vi "Open Swerve Drive.vi"   [LabVIEW 2014]
doc: "Opens references and stores refnums for all swerve drive motors, steering encoders, and gyro(s). The gyros are opened using the Apple Pi gyro library. If you wish to use the normal (WPILib) gyro code, then remove the open blocks from inside this VI."
uses:
  <vilib>/Rock Robotics/SystemInterfaces/DIO/FPGA_DIOPWMChannel.ctl
  <vilib>/Rock Robotics/SystemInterfaces/AI/FPGA_AIChannel.ctl
  <vilib>/Rock Robotics/WPI/MotorControl/WPI_MotorControlOpen Talon.vi
  Global Variables/Refnum Names.vi
types:
  T1 = typedef "FPGA_AIChannel.ctl" = enum8{"AI 0", "AI 1", "AI 2", "AI 3", "AI MXP 0", "AI MXP 1", "AI MXP 2", "AI MXP 3", "Invalid"}
  T2 = typedef "FPGA_DIOPWMChannel.ctl" = enum8{"PWM 0", "PWM 1", "PWM 2", "PWM 3", "PWM 4", "PWM 5", "PWM 6", "PWM 7", "PWM 8", "PWM 9", "PWM MXP 0", "PWM MXP 1", "PWM MXP 2", "PWM MXP 3", "PWM MXP 4", "PWM MXP 5", "PWM MXP 6", "PWM MXP 7", "PWM MXP 8", "PWM MXP 9", "Invalid"}
  T3 = typedef "WPI_MotorControlDeviceRef.ctl" = cluster{"DeviceStatus":errorcluster, "Type":T4, "PWM":cluster{"Controller":T5, "PWM Channel":T2, "DeadBand":T6}, "CAN":cluster{"Device Number":u8, "Control Mode":T7, "Semaphore":T8, "Max Vout":dbl, "TalonSRX Control Mode":T9}, "Invert":bool, "TransformRef":T10, "InvTransformRef":T10}
  T4 = typedef "WPI_MotorControlType.ctl" = enum16{"PWM", "CAN", "CANTalonSRX"}
  T5 = typedef "FPGA_TypedefDigitalModule.ctl" = enum16{"Controller 1"}
  T6 = typedef "WPI_PWMDeadband.ctl" = cluster{"Name":string, "maxPositivePwm":i32, "minPositivePwm":i32, "centerPwm":i32, "maxNegativePwm":i32, "minNegativePwm":i32, "angularRange":u16}
  T7 = typedef "WPI_CANJaguar_ControlMode.ctl" = enum8{"Percent VBus", "Current", "Speed", "Position", "Voltage"}
  T8 = typedef "Semaphore RefNum" = refnum<k1>
  T9 = typedef "WPI_CANTalonSRX_APIControlMode.ctl" = enum8{"Percent VBus", "Speed", "Position", "Slave", "Unchanged / Invalid"}
  T10 = typedef "WPI_PWMTransform_ConPane.ctl" = refnum<vi>
  T11 = typedef "Swerve Sensors DevRef.ctl" = cluster{"Front Right Wheel":T12, "Front Left Wheel":T12, "Rear Right Wheel":T12, "Rear Left Wheel":T12}
  T12 = typedef "WPI_AnalogChannelDevRef.ctl" = cluster{"DevStatus":errorcluster, "Controller":T13, "Analog Channel":T1}
  T13 = typedef "FPGA_TypedefAnalogModule.ctl" = enum16{"Controller 1"}
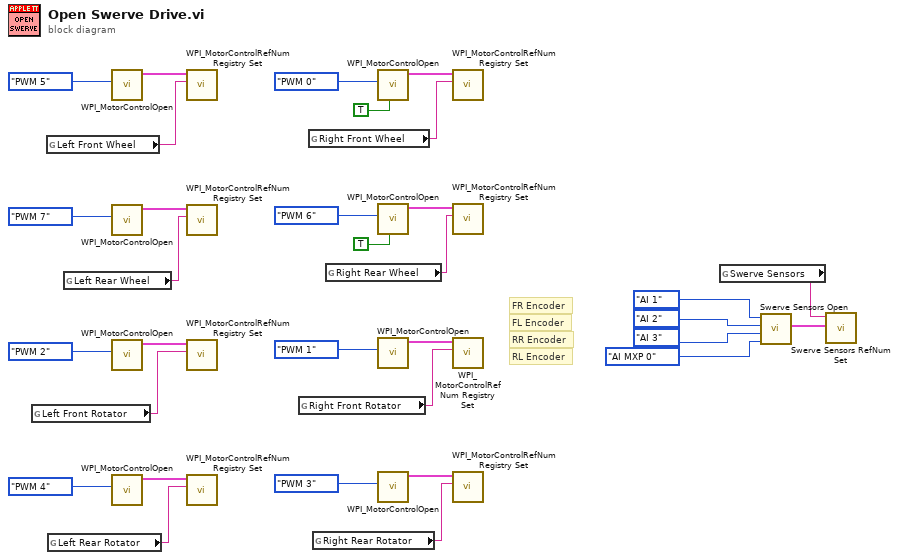
[diagram p0: block diagram]
diagram:
  # "RL Encoder"
  # "RR Encoder"
  # "FL Encoder"
  # "FR Encoder"
  n1 = global read "Refnum Names.vi" "Left Front Rotator"() -> (w7:string)
  n2 = global read "Refnum Names.vi" "Left Front Wheel"() -> (w11:string)
  n3 = global read "Refnum Names.vi" "Left Rear Rotator"() -> (w5:string)
  n4 = global read "Refnum Names.vi" "Left Rear Wheel"() -> (w9:string)
  n5 = call-poly <vilib>:"WPI_MotorControlOpen.vi"("PWM Channel"=FPGA_DIOPWMChannel."PWM 5" ("BL Wheel")) -> ("MotorControlDeviceRef"=w32:T3)  [unwired: 9 in, 1 out]
  n6 = call-poly <vilib>:"WPI_MotorControlOpen.vi"("PWM Channel"=FPGA_DIOPWMChannel."PWM 7" ("BL Spin")) -> ("MotorControlDeviceRef"=w29:T3)  [unwired: 9 in, 1 out]
  n7 = call-poly <vilib>:"WPI_MotorControlOpen.vi"("PWM Channel"=FPGA_DIOPWMChannel."PWM 2" ("BR Wheel")) -> ("MotorControlDeviceRef"=w28:T3)  [unwired: 9 in, 1 out]
  n8 = call-poly <vilib>:"WPI_MotorControlOpen.vi"("PWM Channel"=FPGA_DIOPWMChannel."PWM 4" ("BR Spin")) -> ("MotorControlDeviceRef"=w25:T3)  [unwired: 9 in, 1 out]
  n9 = call <vilib>:"WPI_MotorControlRefNum Registry Set.vi"("refnum name"=w11, "MotorControlDevRef"=w32) -> ()  [unwired: 8 in, 2 out]
  n10 = call <vilib>:"WPI_MotorControlRefNum Registry Set.vi"("refnum name"=w9, "MotorControlDevRef"=w29) -> ()  [unwired: 8 in, 2 out]
  n11 = call <vilib>:"WPI_MotorControlRefNum Registry Set.vi"("refnum name"=w7, "MotorControlDevRef"=w28) -> ()  [unwired: 8 in, 2 out]
  n12 = call <vilib>:"WPI_MotorControlRefNum Registry Set.vi"("refnum name"=w5, "MotorControlDevRef"=w25) -> ()  [unwired: 8 in, 2 out]
  n13 = global read "Refnum Names.vi" "Right Front Rotator"() -> (w6:string)
  n14 = global read "Refnum Names.vi" "Right Front Wheel"() -> (w10:string)
  n15 = global read "Refnum Names.vi" "Right Rear Rotator"() -> (w4:string)
  n16 = global read "Refnum Names.vi" "Right Rear Wheel"() -> (w8:string)
  n17 = call-poly <vilib>:"WPI_MotorControlOpen.vi"("Invert"=TRUE, "PWM Channel"=FPGA_DIOPWMChannel."PWM 0" ("FL Wheel")) -> ("MotorControlDeviceRef"=w24:T3)  [unwired: 8 in, 1 out]
  n18 = call-poly <vilib>:"WPI_MotorControlOpen.vi"("Invert"=TRUE, "PWM Channel"=FPGA_DIOPWMChannel."PWM 6" ("FL Spin")) -> ("MotorControlDeviceRef"=w21:T3)  [unwired: 8 in, 1 out]
  n19 = call-poly <vilib>:"WPI_MotorControlOpen.vi"("PWM Channel"=FPGA_DIOPWMChannel."PWM 1" ("FR Wheel")) -> ("MotorControlDeviceRef"=w20:T3)  [unwired: 9 in, 1 out]
  n20 = call-poly <vilib>:"WPI_MotorControlOpen.vi"("PWM Channel"=FPGA_DIOPWMChannel."PWM 3" ("FR Spin")) -> ("MotorControlDeviceRef"=w17:T3)  [unwired: 9 in, 1 out]
  n21 = call <vilib>:"WPI_MotorControlRefNum Registry Set.vi"("refnum name"=w10, "MotorControlDevRef"=w24) -> ()  [unwired: 8 in, 2 out]
  n22 = call <vilib>:"WPI_MotorControlRefNum Registry Set.vi"("refnum name"=w8, "MotorControlDevRef"=w21) -> ()  [unwired: 8 in, 2 out]
  n23 = call <vilib>:"WPI_MotorControlRefNum Registry Set.vi"("refnum name"=w6, "MotorControlDevRef"=w20) -> ()  [unwired: 8 in, 2 out]
  n24 = call <vilib>:"WPI_MotorControlRefNum Registry Set.vi"("refnum name"=w4, "MotorControlDevRef"=w17) -> ()  [unwired: 8 in, 2 out]
  n25 = global read "Refnum Names.vi" "Swerve Sensors"() -> (w3:string)
  n26 = call "Swerve Sensors Open.vi"("Rear Left Wheel"=FPGA_AIChannel."AI MXP 0", "Rear Right Wheel"=FPGA_AIChannel."AI 3", "Front Left Wheel"=FPGA_AIChannel."AI 2", "Front Right Wheel"=FPGA_AIChannel."AI 1") -> ("Swerve Sensors DevRef"=w12:T11)  [unwired: 7 in]
  n27 = call "Swerve Sensors RefNum Set.vi"("Swerve Sensors DevRef"=w12, "Swerve Sensors Name"=w3) -> ()  [unwired: 10 in]
